vi "Initialise.vi"(5 "Initial Position":T1={"x"=500.0, "y"=500.0}, 6 "Acceleration [m/s/s]":sgl=10.0 format="%.3g", 7 "Field Size":T1={"x"=500.0, "y"=500.0}, 8 "Maximum Velocity [m/s]":sgl=10.0 format="%.3g", 9 "Turn Rate [deg/s]":sgl=90.0 format="%.3g", 10 "Initial Heading [deg]":sgl=45.0 format="%#_13g", 11 "Initial Velocity [m/s]":sgl=1.0 format="%#_13g") -> (3 "Motion out":refnum<class "Motion.lvclass">)   [LabVIEW 2021, in "Motion.lvclass"]
uses:
  Motion.lvclass
  Re-use Libraries/Vector 2D/Vector 2D.lvclass
  Motion.lvclass/Motion.ctl
  Math/Vec2.ctl
  Math/Math.lvlib
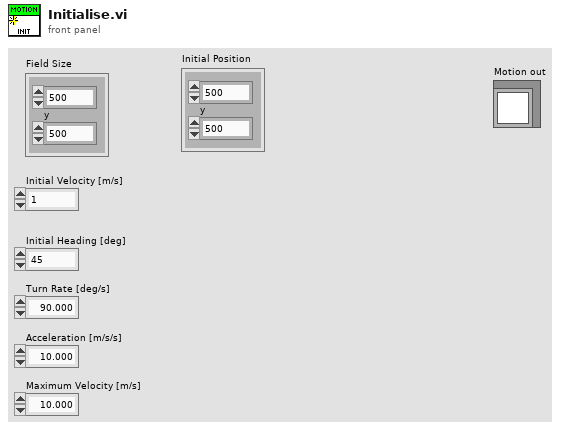
[diagram p1: front panel]
types:
  T1 = typedef "Math.lvlib/Vec2.ctl" = cluster{"x":sgl, "y":sgl}
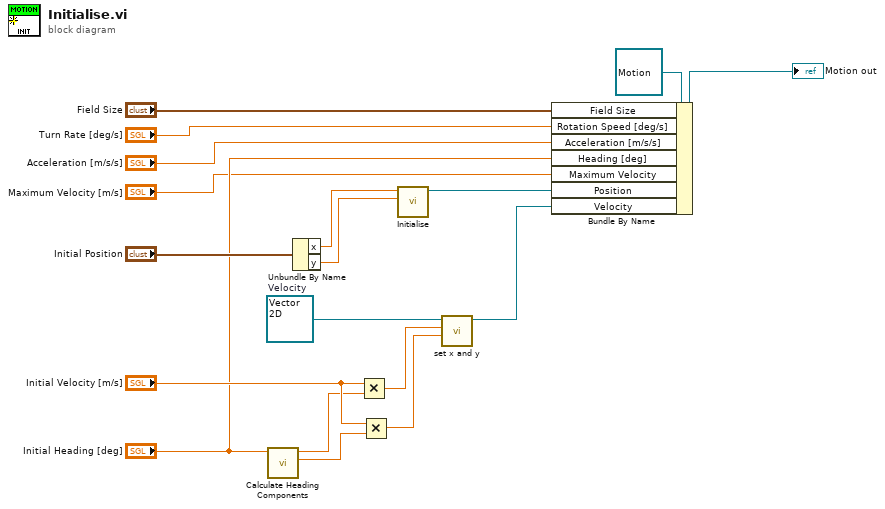
[diagram p0: block diagram]
diagram:
  w14 = refnum<class "Vector 2D.lvclass"> refnum  # Velocity
  n1 = call "Calculate Heading Components.vi"("Heading In [deg]"="Initial Heading [deg]") -> ("Sin Heading"=w8:sgl, "Cos Heading"=w9:sgl)  [unwired: 9 in]
  n2 = Unbundle By Name("Initial Position") -> ("x"=w4:sgl, "y"=w3:sgl)
  n3 = Multiply(x="Initial Velocity [m/s]", y=w9) -> (x*y=w15:sgl)
  n4 = Multiply(x="Initial Velocity [m/s]", y=w8) -> (x*y=w16:sgl)
  n5 = call "Initialise.vi"("y"=w3, "x"=w4) -> ("Vector 2D out"=w2:refnum<class "Vector 2D.lvclass">)  [unwired: 9 in]
  n6 = call "set x and y.vi"("y"=w16, "x"=w15, "Vector 2D in"=w14) -> ("Vector 2D out"=w10:refnum<class "Vector 2D.lvclass">)  [unwired: 8 in]
  n7 = Bundle By Name(cluster=refnum<class "Motion.lvclass"> refnum ("Motion in"), "Field Size"="Field Size", "Rotation Speed [deg/s]"="Turn Rate [deg/s]", "Acceleration [m/s/s]"="Acceleration [m/s/s]", "Heading [deg]"="Initial Heading [deg]", "Maximum Velocity"="Maximum Velocity [m/s]", "Position"=w2, "Velocity"=w10) -> (→"Motion out":refnum<class "Motion.lvclass">)
